vi "数据库提取IOTdata.vi"() -> (0 "in spec?":bool, 1 "data":string[](array[string]), 2 "次数&压力":string[](array[string]), 3 "SN":string)   [LabVIEW 2017]
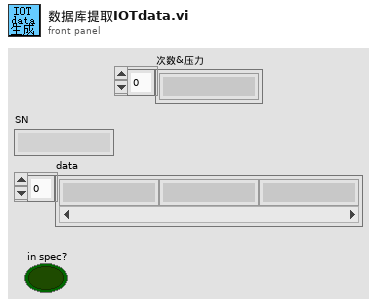
[diagram p1: front panel]
types:
  T1 = typedef "IOTdata集合.ctl" = cluster{"p300data":T2, "p400data":T2, "p100data":string[][], "p200data":string[][], "对位次数&压力":cluster{"对位次数":dbl, "压力":dbl}}
  T2 = typedef "P300&P400结果.ctl" = cluster{"对位结果":string[][], "DX":bool, "DY":bool, "Y3-Y4":bool}
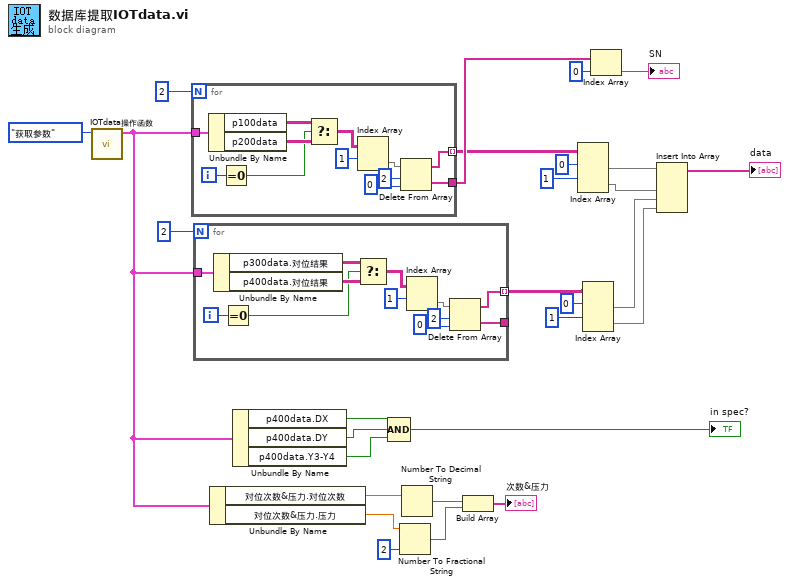
[diagram p0: block diagram]
diagram:
  n1 = call "IOTdata操作函数.vi"("操作选项"=enum16{"初始化", "获取参数", "写入参数"}."获取参数") -> ("IOTdata集合"=w7:T1)  [unwired: 10 in]
  n2 = for {
    N: 2 -> [_]
    tunnel: w7 -> [w36]
    tunnel: [w30] -> w26
    tunnel: [w29] -> w22 mode=indexing
    i -> [w35]
    n3 = Unbundle By Name(w36) -> ("p100data"=w34:string[][], "p200data"=w33:string[][])
    n4 = Equal To 0?(x=w35) -> (x = 0?=w32:bool)
    n5 = Select(t=w34, s=w32, f=w33) -> (s? t:f=w31:string[][])
    n6 = Index Array(array=w31, index (row)=1 ("索引 (行)")) -> (element=w39:string[])  [unwired: 1 in]
    n7 = Delete From Array(array=w39, length=2 ("长度"), index=0 ("长度")) -> (deleted portion=w30:string[], array with subset deleted=w29:string[])
  }
  n8 = for {
    N: 2 -> [_]
    tunnel: w7 -> [w48]
    tunnel: [w42] -> _
    tunnel: [w41] -> w17 mode=indexing
    i -> [w47]
    n9 = Unbundle By Name(w48) -> ("p300data.对位结果"=w46:string[][], "p400data.对位结果"=w45:string[][])
    n10 = Equal To 0?(x=w47) -> (x = 0?=w44:bool)
    n11 = Select(t=w46, s=w44, f=w45) -> (s? t:f=w43:string[][])
    n12 = Index Array(array=w43, index (row)=1 ("索引 (行)")) -> (element=w51:string[])  [unwired: 1 in]
    n13 = Delete From Array(array=w51, length=2 ("长度"), index=0 ("长度")) -> (deleted portion=w42:string[], array with subset deleted=w41:string[])
  }
  n14 = Unbundle By Name(w7) -> ("对位次数&压力.对位次数"=w6:dbl, "对位次数&压力.压力"=w5:dbl)
  n15 = Unbundle By Name(w7) -> ("p400data.DX"=w11:bool, "p400data.DY"=w10:bool, "p400data.Y3-Y4"=w9:bool)
  n16 = Compound Arithmetic op=AND ("复合运算")(w11, w10, w9) -> (→"in spec?":bool)
  n17 = Number To Fractional String(number=w5, precision (6)=i16 2 ("精度(6)")) -> (F-format string=w2:string)  [unwired: 2 in]
  n18 = Number To Decimal String(number=w6) -> (decimal integer string=w3:string)  [unwired: 1 in]
  n19 = Build Array(w3, w2) -> (→"次数&压力":string[])
  n20 = Index Array(array=w22, index (row) #1=0 ("索引 (行)"), index (row) #2=1 ("索引 (行)")) -> (element #1=w16:string[], element #2=w15:string[])  [unwired: 2 in]
  n21 = Index Array(array=w17, index (row) #1=0 ("索引 (行)"), index (row) #2=1 ("索引 (行)")) -> (element #1=w14:string[], element #2=w13:string[])  [unwired: 2 in]
  n22 = Index Array(array=w26, index=0 ("索引")) -> (element=→"SN":string)
  n23 = Insert Into Array(array=w16, new element #1=w15, new element #2=w14, new element #3=w13) -> (→"data":string[])  [unwired: 1 in]
